vi "Multiply Class Test.vi"(11 "Error In":errorcluster) -> (15 "Error Out":errorcluster)   [LabVIEW 2021, in "Test Files.lvlib"]
doc: "This VI has test cases for checking the functionality of multiply class using caraya unit test framework."
uses:
  Test Files.lvlib
  <vilib>/addons/_JKI Toolkits/Caraya/classes/Test/Test.lvclass
  <vilib>/addons/_JKI Toolkits/Caraya/classes/Assert/Assert.lvclass
  Classes/NumericOperation/NumericOperation.lvclass
  Controls/Test Data Cluster.ctl
  <vilib>/addons/_JKI Toolkits/Caraya/classes/Assert/Assert Equal Value_Variant.vi
panel:
  # "Multiply Class Test"
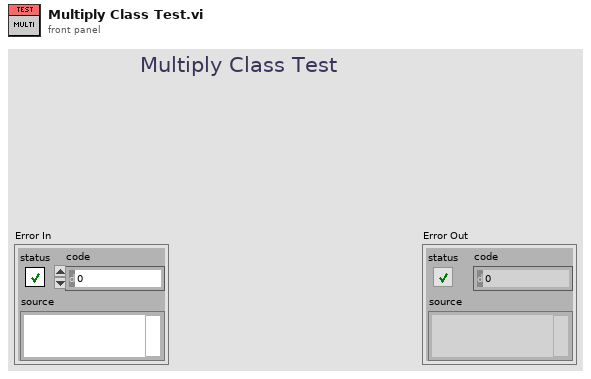
[diagram p1: front panel]
types:
  T1 = typedef "Test Data Cluster.ctl" = cluster{"A":dbl, "B":dbl, "Output":dbl}
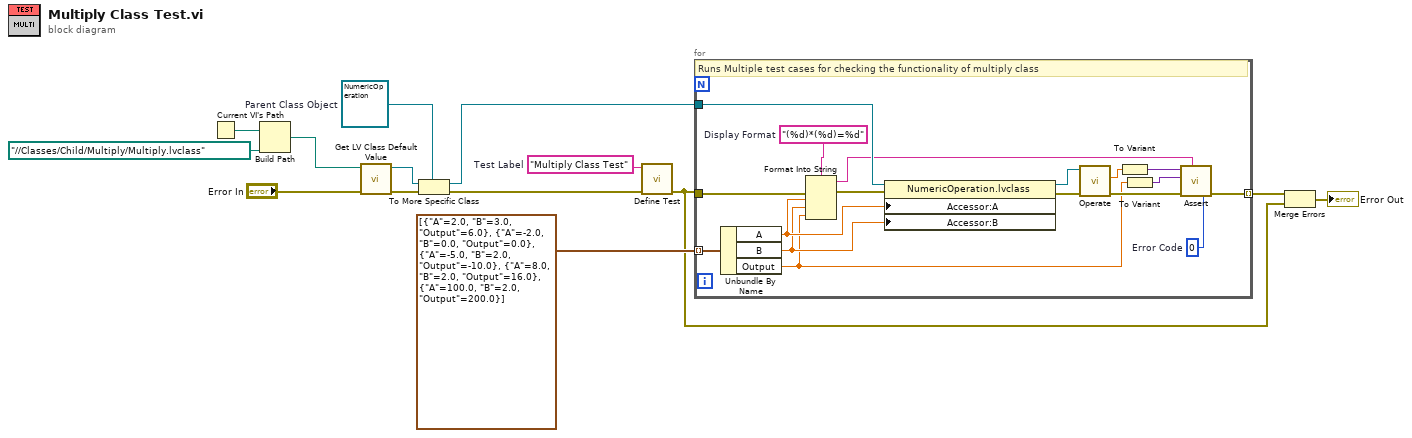
[diagram p0: block diagram]
diagram:
  w7 = refnum<class "NumericOperation.lvclass"> refnum  # Parent Class Object
  w8 = "Multiply Class Test"  # Test Label
  n1 = Current VI's Path() -> (path=w14:path)
  n2 = Build Path(base path=w14, name or relative path=path "../../Classes/Child/Multiply/Multiply.lvclass") -> (appended path=w12:path)
  n3 = call <vilib>:"Get LV Class Default Value.vi"("error in (no error)"="Error In", "class path"=w12) -> ("error out"=w10:errorcluster, "object"=w6:refnum<class>)  [unwired: 8 in]
  n4 = To More Specific Class(target class=w7, reference=w6, error in=w10) -> (specific class reference=w5:refnum<class "NumericOperation.lvclass">, error out=w9:errorcluster)
  n5 = call <vilib>:"Define Test.vi"("error in (no error)"=w9, "Label (VI Title)"=w8) -> ("error out"=w1:errorcluster)  [unwired: 8 in, 1 out]
  n6 = for {
    tunnel: w5 -> [w28]
    tunnel: T1[] [{"A"=2.0, "B"=3.0, "Output"=6.0}, {"A"=-2.0, "B"=0.0, "Output"=0.0}, {"A"=-5.0, "B"=2.0, "Output"=-10.0}, {"A"=8.0, "B"=2.0, "Output"=16.0}, {"A"=100.0, "B"=2.0, "Output"=200.0}] -> [w27] mode=indexing
    tunnel: w1 -> [w31]
    tunnel: [w20] -> w2 mode=indexing
    w18 = 0  # Error Code
    w30 = "(%d)*(%d)=%d"  # Display Format
    # "Runs Multiple test cases for checking the functionality of multiply class"
    n7 = Unbundle By Name(w27) -> ("A"=w17:dbl, "B"=w16:dbl, "Output"=w15:dbl)
    n8 = Format Into String(format string=w30, error in=w31, w17, w16, w15) -> (resulting string=w19:string, error out=w29:errorcluster)  [unwired: 1 in]
    n9 = property class="NumericOperation.lvclass"(reference=w28, error in=w29, "Accessor:A"=w17, "Accessor:B"=w16) -> (reference out=w25:refnum<class "NumericOperation.lvclass">, error out=w26:errorcluster)
    n10 = call-dynamic "Operate.vi"("error in (no error)"=w26, "NumericOperation in"=w25) -> ("error out"=w21:errorcluster, "C"=w24:dbl)  [unwired: 7 in, 1 out]
    n11 = To Variant(anything=w24) -> (Variant=w23:variant)
    n12 = To Variant(anything=w15) -> (Variant=w22:variant)
    n13 = call-poly <vilib>:"Assert.vi"("error code (1)"=w18, "Label"=w19, "error in (no error)"=w21, "Y"=w22, "X"=w23) -> ("error out"=w20:errorcluster)  [unwired: 5 in, 1 out]
  }
  n14 = Merge Errors(w2, w1) -> (→"Error Out":errorcluster)
